vi "PreviewMessage.vi"() -> ()   [LabVIEW 2015]
uses:
  TypeDefs/MessageCluster.ctl
panel:
  in  "error in (no error)":errorcluster
  out "error out":errorcluster
  out "dupMessageQueue":refnum<queue>
  in  "MessageQueue":refnum<queue>
  out "Message":string
  out "MessageData":variant
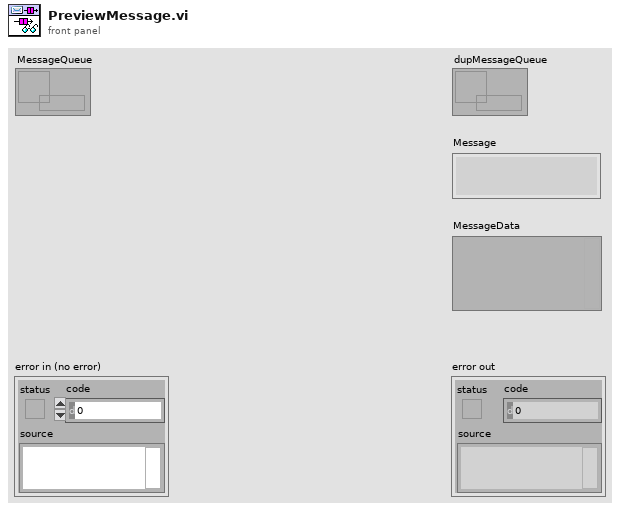
[diagram p1: front panel]
types:
  T1 = typedef "MessageCluster.ctl" = cluster{"Message":string, "MessageData":variant}
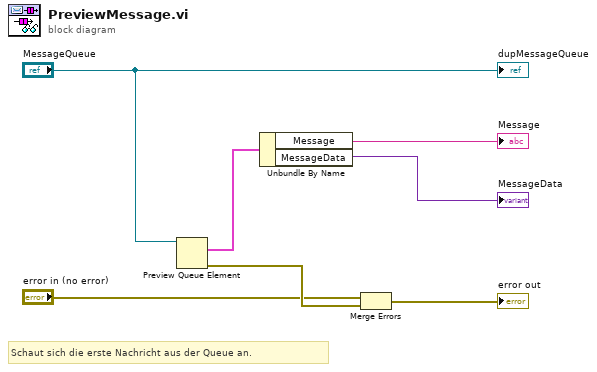
[diagram p0: block diagram]
diagram:
  # "Schaut sich die erste Nachricht aus der Queue an."
  n1 = Preview Queue Element(queue="MessageQueue") -> (element=w4:T1, error out=w7:errorcluster)  [unwired: 2 in, 2 out]
  n2 = Unbundle By Name(w4) -> ("Message"=→"Message":string, "MessageData"=→"MessageData":variant)
  n3 = Merge Errors("error in (no error)", w7) -> (→"error out":errorcluster)
  "dupMessageQueue" <- "MessageQueue"
